vi "LoadProfilePowerTestK2.vi"() -> ()   [LabVIEW 2020]
uses:
  <instrlib>/NH Research Regenerative Test Series/Public/Configure/Output Safety.ctl
  <vilib>/DAQmx/read.llb/DAQmx Read (Analog 1D DBL NChan 1Samp).vi
  <instrlib>/NH Research Regenerative Test Series/Public/Data/Read (Ave Current).vi
  <instrlib>/NH Research Regenerative Test Series/Public/Data/Low Level/Fetch (Ave Voltage).vi
  <instrlib>/NH Research Regenerative Test Series/Public/Data/Low Level/Fetch (Ave True Power).vi
  <vilib>/DAQmx/miscellaneous.llb/DAQmx Fill In Error Info.vi
  <instrlib>/NH Research Regenerative Test Series/NH Research Regenerative Test Series.lvlib
panel:
  in  "Starting Charge State (%)":dbl format="%#.6g"
  in  "Starting Cycle life":dbl format="%#.6g"
  out "Remaining Cycle life":dbl
  out "DoD":dbl
  in  "Battery Capacity (Wh)":dbl format="%#.6g"
  out "Total Power":dbl
  out "Current Step":dbl
  out "Time  Elapsed":dbl
  out "Time Step":dbl
  out "Load Output (A)":dbl
  out "Time Ref":dbl
  out "Control Power":dbl
  in  "Time Array":dbl[](array[numeric])
  in  "Power":dbl[](array[numeric])
  in  "Test Time (s)":dbl format="%#.6g"
  out "BatteryTempInternal":dbl
  out "BatteryTempExt":dbl
  out "BatteryWaterOut":dbl
  out "BatteryWaterIn":dbl
  out "Task error out":errorcluster
  out "String":string
  in  "Output Safety":T1
  out "Filename Out":path
  in  "DAQmx Task Name":refnum<k21>
  in  "Path":path
  out "Ave Current (A)":dbl
  out "Ave Voltage (V)":dbl
  out "Ave True Power (W)":dbl
  out "Status Byte Register":T2
  in  "Logical Instrument Number":u32=1
  in  "Voltage Setpoint (0 V)":dbl format="%#.6g"
  in  "Battery Detect Voltage (0V)":dbl format="%#.6g"
  in  "VISA resource name":refnum<visa-resource-name>
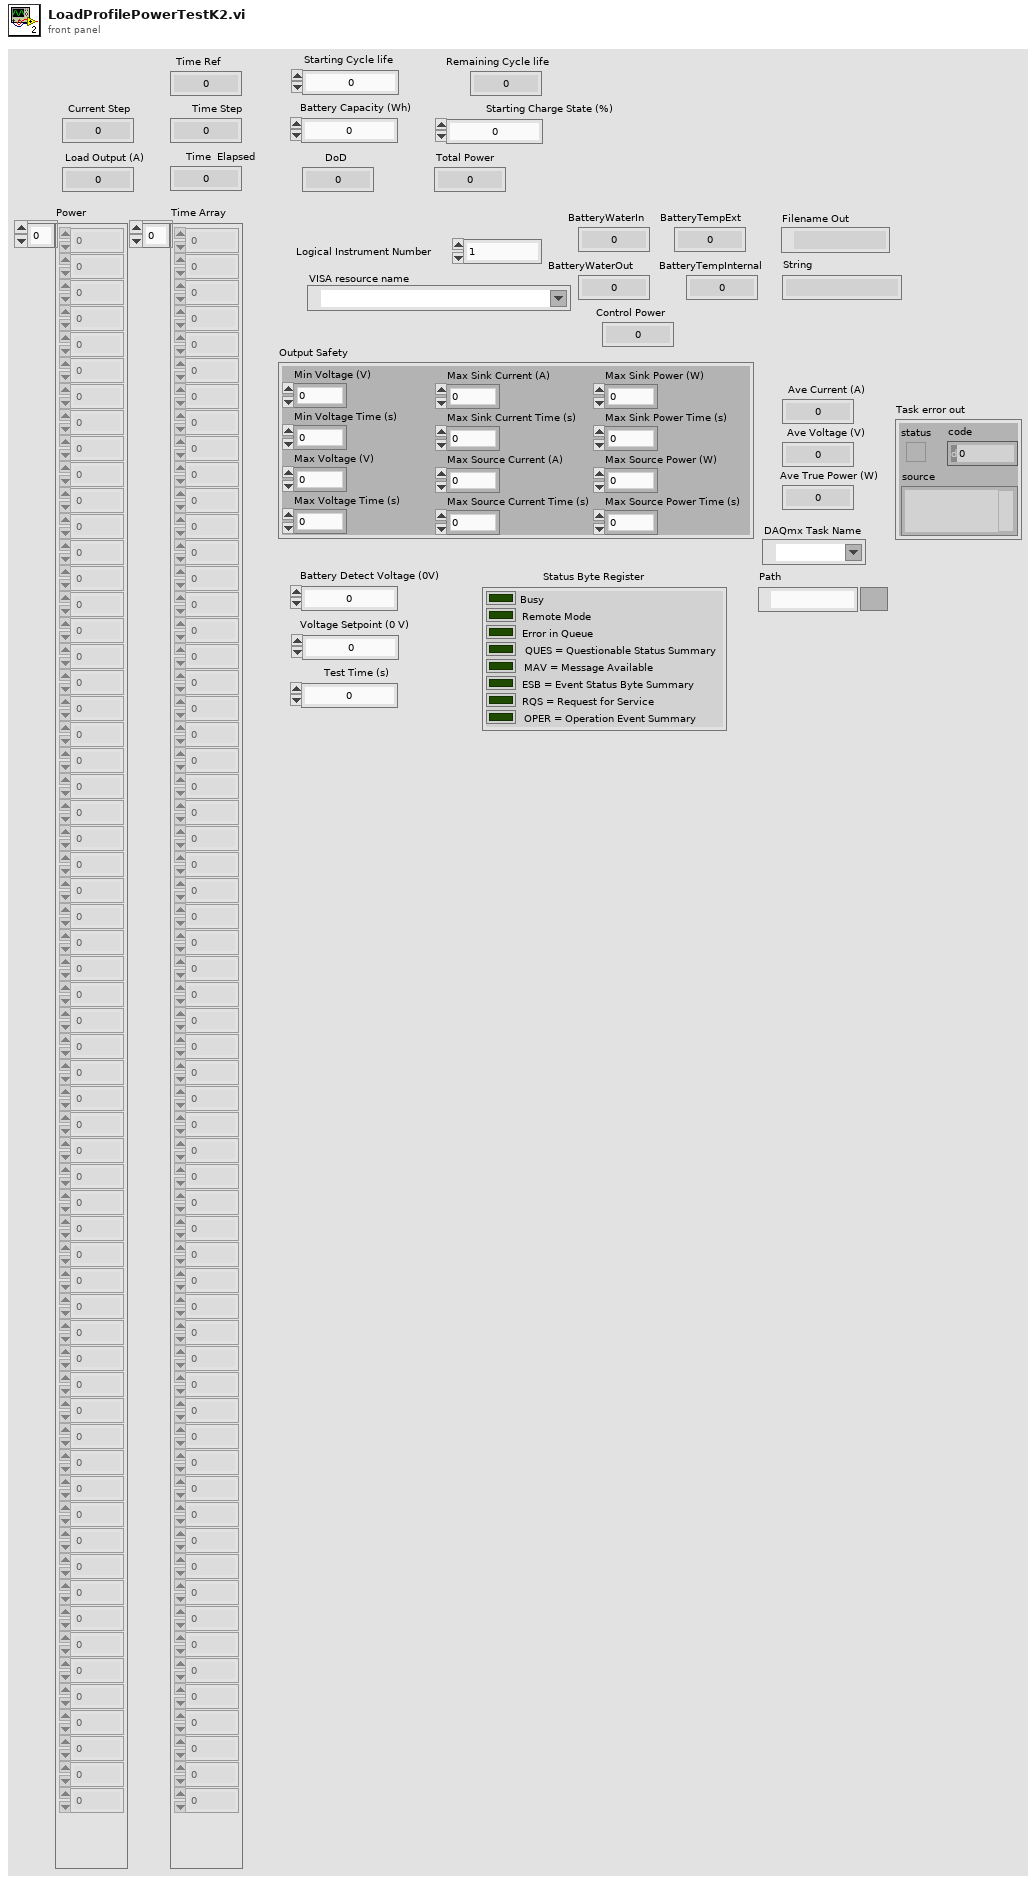
[diagram p1: front panel]
types:
  T1 = typedef "NH Research Regenerative Test Series.lvlib/Output Safety.ctl" = cluster{"Min Voltage (V)":dbl, "Min Voltage Time (s)":dbl, "Max Voltage (V)":dbl, "Max Voltage Time (s)":dbl, "Max Sink Current (A)":dbl, "Max Sink Current Time (s)":dbl, "Max Source Current (A)":dbl, "Max Source Current Time (s)":dbl, "Max Sink Power (W)":dbl, "Max Sink Power Time (s)":dbl, "Max Source Power (W)":dbl, "Max Source Power Time (s)":dbl}
  T2 = cluster{"Busy":bool, "Remote Mode":bool, "Error in Queue":bool, "QUES = Questionable Status Summary":bool, "MAV = Message Available":bool, "ESB = Event Status Byte Summary":bool, "RQS = Request for Service":bool, "OPER = Operation Event Summary":bool}
  T3 = cluster{"data[0]":dbl, "data[1]":dbl, "data[2]":dbl, "data[3]":dbl, "data[4]":dbl, "data[5]":dbl, "data[6]":dbl, "data[7]":dbl, "data[8]":dbl}
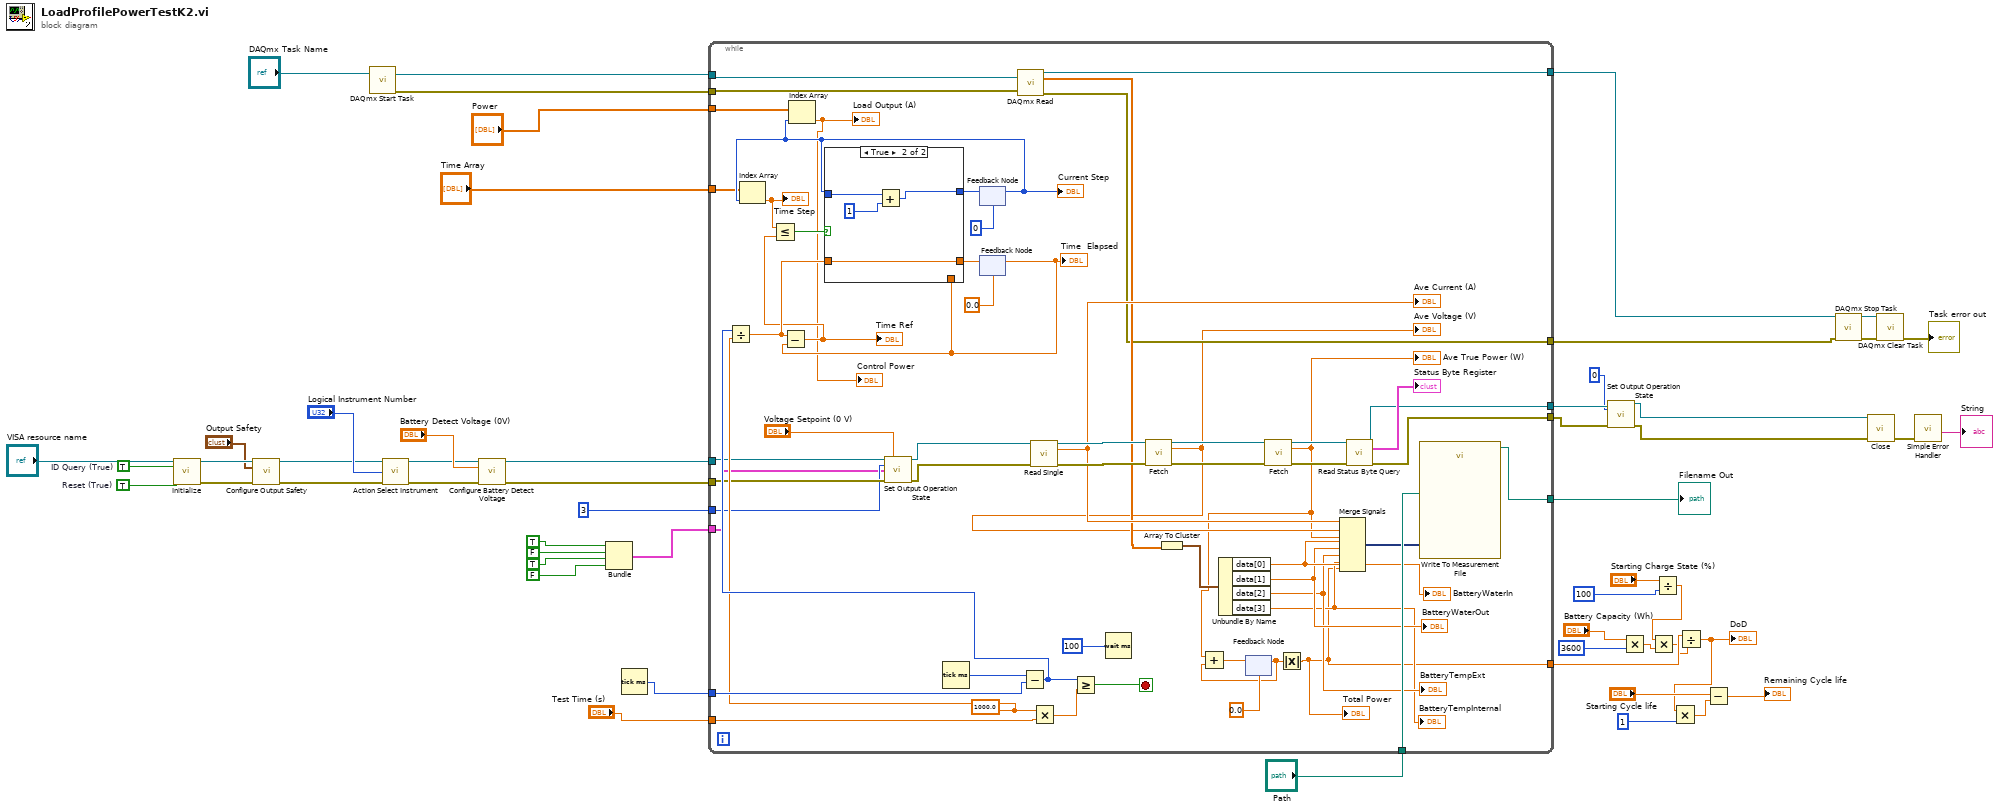
[diagram p0: block diagram]
diagram:
  w48 = TRUE  # ID Query (True)
  w47 = TRUE  # Reset (True)
  n1 = call <vilib>:"Initialize.vi"("VISA resource name"="VISA resource name", "ID Query (True)"=w48, "Reset (True)"=w47) -> ("VISA resource name out"=w46:refnum<visa-resource-name>, "error out"=w45:errorcluster)  [unwired: 11 in]
  n2 = call <vilib>:"Configure Output Safety.vi"("VISA resource name"=w46, "Output Safety"="Output Safety", "error in (no error)"=w45) -> ("VISA resource name out"=w42:refnum<visa-resource-name>, "error out"=w31:errorcluster)  [unwired: 11 in]
  n3 = call <vilib>:"DAQmx Start Task.vi"("task/channels in"="DAQmx Task Name") -> ("task out"=w40:refnum<k21>, "error out"=w32:errorcluster)  [unwired: 13 in]
  n4 = call <instrlib>:"Action Select Instrument.vi"("VISA resource name"=w42, "Logical Instrument Number"="Logical Instrument Number", "error in (no error)"=w31) -> ("VISA resource name out"=w53:refnum<visa-resource-name>, "error out"=w52:errorcluster)  [unwired: 11 in]
  n5 = call <vilib>:"Configure Battery Detect Voltage.vi"("VISA resource name"=w53, "Battery Detect Voltage (0V)"="Battery Detect Voltage (0V)", "error in (no error)"=w52) -> ("VISA resource name out"=w29:refnum<visa-resource-name>, "error out"=w28:errorcluster)  [unwired: 11 in]
  n6 = Bundle(TRUE, FALSE, TRUE, FALSE) -> (w23:cluster{bool, bool, bool, bool})  [unwired: 1 in]
  n7 = Tick Count (ms)() -> (millisecond timer value=w30:u32)
  n8 = while {
    tunnel: [w104] -> w5
    tunnel: [w103] -> w3
    tunnel: "Path" -> [w101]
    tunnel: w40 -> [w100]
    tunnel: [w96] -> w34
    tunnel: [w95] -> w33
    tunnel: w32 -> [w94]
    tunnel: [w93] -> w49
    tunnel: w30 -> [w85]
    tunnel: "Test Time (s)" -> [w84]
    tunnel: w29 -> [w59]
    tunnel: w28 -> [w58]
    tunnel: w23 -> [w56]
    tunnel: 3 -> [w57]
    tunnel: "Power" -> [w71]
    tunnel: "Time Array" -> [w70]
    tunnel: [w63] -> w16
    stop <- w83 stop-if-true
    w68 = 1000.0
    n9 = call <vilib>:"Set Output Operation State.vi"("VISA resource name"=w59, "Voltage Setpoint (0 V)"="Voltage Setpoint (0 V)", "Mode (0: Off)"=w57, "Enable"=w56, "error in (no error)"=w58) -> ("VISA resource name out"=w61:refnum<visa-resource-name>, "error out"=w55:errorcluster)  [unwired: 9 in]
    n10 = Tick Count (ms)() -> (millisecond timer value=w86:u32)
    n11 = feedback #1(0) -> (w72:i32)
    "Current Step" <- w72
    n12 = Index Array(array=w70, index=w72) -> (element=w69:dbl)
    "Time Step" <- w69
    n13 = Index Array(array=w71, index=w72) -> (element=→"Control Power" →"Load Output (A)":dbl)
    n14 = feedback #2(0.0) -> (w80:dbl)
    "Time  Elapsed" <- w80
    n15 = call-poly <vilib>:"DAQmx Read.vi"("task/channels in"=w100, "error in"=w94) -> ("task out"=w96:refnum<k21>, "data"=w99:dbl[], "error out"=w95:errorcluster)  [unwired: 11 in]
    n16 = Subtract(x=w86, y=w85) -> (x-y=w74:u32)
    n17 = Divide(x=w74, y=w68) -> (x/y=w82:dbl)
    n18 = Subtract(x=w82, y=w80) -> (x-y=w77:dbl)
    "Time Ref" <- w77
    n19 = Less Or Equal?(x=w69, y=w77) -> (x <= y?=w78:bool)
    n20 = case shown="True" w78 {
      tunnel: w82 -> [_ w117]
      tunnel: [w113 w117] -> w81
      tunnel: w80 -> [w113 _]
      tunnel: [w112 w115] -> w79
      tunnel: w72 -> [w112 w114]
      frame False {
      }
      frame True {
        n21 = Add(x=w114, y=1) -> (x+y=w115:i32)
      }
    }
    n22 = feedback-in #1(w79) -> ()
    n23 = feedback-in #2(w81) -> ()
    n24 = call-poly <instrlib>:"Read Single.vi"("VISA resource name"=w61, "error in (no error)"=w55) -> ("VISA resource name out"=w110:refnum<visa-resource-name>, "Ave Current (A)"=w102:dbl, "error out"=w111:errorcluster)  [unwired: 11 in]
    "Ave Current (A)" <- w102
    n25 = Multiply(x=w68, y=w84) -> (x*y=w73:dbl)
    n26 = Greater Or Equal?(x=w74, y=w73) -> (x >= y?=w83:bool)
    n27 = Wait (ms)(milliseconds to wait=100) -> ()  [unwired: 1 out]
    n28 = call-poly <instrlib>:"Fetch.vi"("VISA resource name"=w110, "error in (no error)"=w111) -> ("VISA resource name out"=w109:refnum<visa-resource-name>, "Ave Voltage (V)"=w92:dbl, "error out"=w108:errorcluster)  [unwired: 11 in]
    "Ave Voltage (V)" <- w92
    n29 = Array To Cluster(array=w99) -> (cluster=w98:T3)
    n30 = Unbundle By Name(w98) -> ("data[0]"=w91:dbl, "data[1]"=w90:dbl, "data[2]"=w89:dbl, "data[3]"=w88:dbl)
    "BatteryWaterIn" <- w91
    "BatteryWaterOut" <- w90
    "BatteryTempExt" <- w89
    "BatteryTempInternal" <- w88
    n31 = feedback #3(0.0) -> (w62:dbl)
    n32 = call-poly <instrlib>:"Fetch.vi"("VISA resource name"=w109, "error in (no error)"=w108) -> ("VISA resource name out"=w107:refnum<visa-resource-name>, "Ave True Power (W)"=w65:dbl, "error out"=w106:errorcluster)  [unwired: 11 in]
    "Ave True Power (W)" <- w65
    n33 = Add(x=w65, y=w62) -> (x+y=w66:dbl)
    n34 = feedback-in #3(w66) -> ()
    n35 = Absolute Value(x=w62) -> (abs(x)=w63:dbl)
    "Total Power" <- w63
    n36 = Merge Signals "Merge Signals"(w102, w92, w65, w91, w90, w89, w88, w63) -> (w97:dynamicdata)
    n37 = call <instrlib>:"Read Status Byte Query.vi"("VISA resource name"=w107, "error in (no error)"=w106) -> ("VISA resource name out"=w104:refnum<visa-resource-name>, "Status Byte Register"=→"Status Byte Register":T2, "error out"=w103:errorcluster)  [unwired: 11 in]
    n38 = call "Write To Measurement File"("Signals"=w97, "Filename"=w101) -> ("Filename Out"=w93:path)  [unwired: 15 in, 2 out]
  }
  "Filename Out" <- w49
  n39 = call <vilib>:"Set Output Operation State.vi"("VISA resource name"=w5, "Mode (0: Off)"=0, "error in (no error)"=w3) -> ("VISA resource name out"=w2:refnum<visa-resource-name>, "error out"=w1:errorcluster)  [unwired: 11 in]
  n40 = Multiply(x="Battery Capacity (Wh)", y=3600) -> (x*y=w7:dbl)
  n41 = Divide(x="Starting Charge State (%)", y=100) -> (x/y=w6:dbl)
  n42 = Multiply(x=w6, y=w7) -> (x*y=w8:dbl)
  n43 = Divide(x=w16, y=w8) -> (x/y=w13:dbl)
  "DoD" <- w13
  n44 = Multiply(x=w13, y=1) -> (x*y=w14:dbl)
  n45 = Subtract(x="Starting Cycle life", y=w14) -> (x-y=→"Remaining Cycle life":dbl)
  n46 = call <vilib>:"DAQmx Stop Task.vi"("task/channels in"=w34, "error in"=w33) -> ("task out"=w38:refnum<k21>, "error out"=w37:errorcluster)  [unwired: 12 in]
  n47 = call <instrlib>:"Close.vi"("VISA resource name"=w2, "error in (no error)"=w1) -> ("error out"=w35:errorcluster)  [unwired: 13 in]
  n48 = call <vilib>:"DAQmx Clear Task.vi"("task in"=w38, "error in"=w37) -> ("error out"=→"Task error out":errorcluster)  [unwired: 13 in]
  n49 = call <vilib>:"Simple Error Handler.vi"("error in (no error)"=w35) -> ("source out"=→"String":string)  [unwired: 4 in, 4 out]
